vi "Teleop Rollers Control.vi"(9 "Driver Buttons":T1, 10 "Manipulator Axes":T2, 11 "Manipulator Buttons":T1) -> (3 "Roller Command":T3)   [LabVIEW 2013]
uses:
  <vilib>/Rock Robotics/WPI/Joystick/WPI_JoystickButtonState.ctl
  Roller Control.ctl
  Roller Mode.ctl
  Common Code/Change Detect Boolean.vi
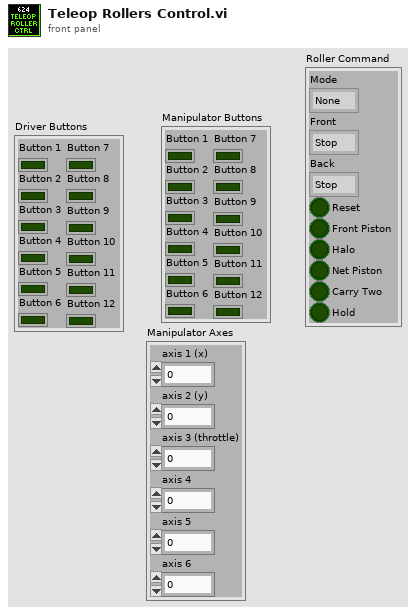
[diagram p1: front panel]
types:
  T1 = typedef "WPI_JoystickButtonState.ctl" = cluster{"Button 1":bool, "Button 2":bool, "Button 3":bool, "Button 4":bool, "Button 5":bool, "Button 6":bool, "Button 7":bool, "Button 8":bool, "Button 9":bool, "Button 10":bool, "Button 11":bool, "Button 12":bool}
  T2 = cluster{"axis 1 (x)":dbl, "axis 2 (y)":dbl, "axis 3 (throttle)":dbl, "axis 4":dbl, "axis 5":dbl, "axis 6":dbl}
  T3 = typedef "Roller Control.ctl" = cluster{"Mode":T4, "Front":enum16{"Stop", "Forward", "Reverse"}, "Back":enum16{"Stop", "Forward", "Reverse"}, "Reset":bool, "Front Piston":bool, "Halo":bool, "Net Piston":bool, "Carry Two":bool, "Hold":bool}
  T4 = typedef "Roller Mode.ctl" = enum16{"None", "Front", "Back", "Both", "Manual"}
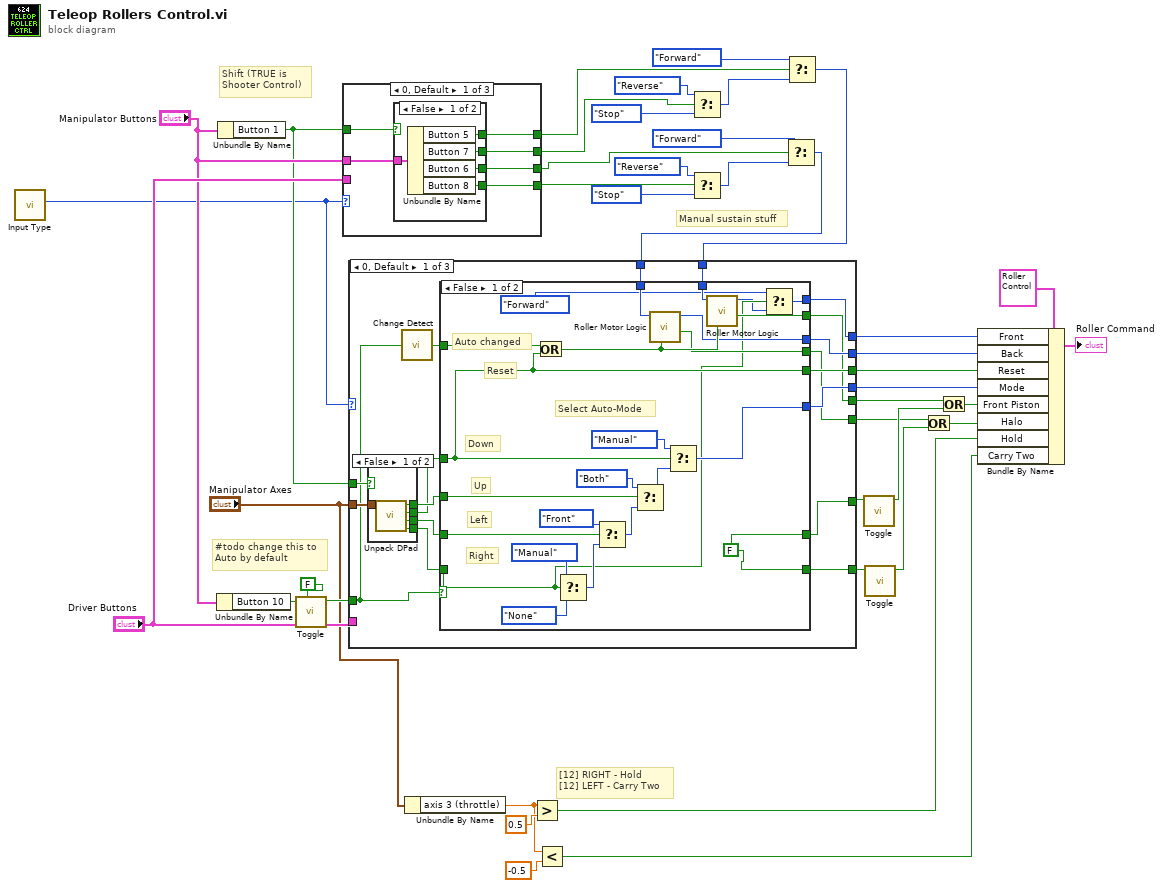
[diagram p0: block diagram]
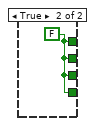
[diagram p2: hidden frame]
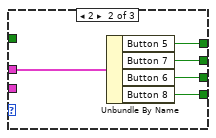
[diagram p3: hidden frame]
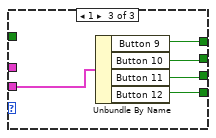
[diagram p4: hidden frame]
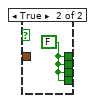
[diagram p5: hidden frame]
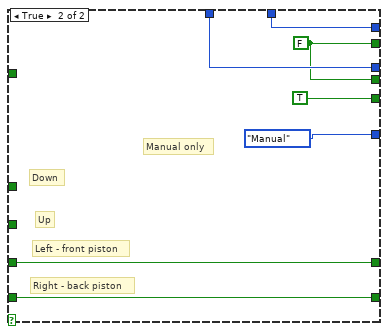
[diagram p6: hidden frame]
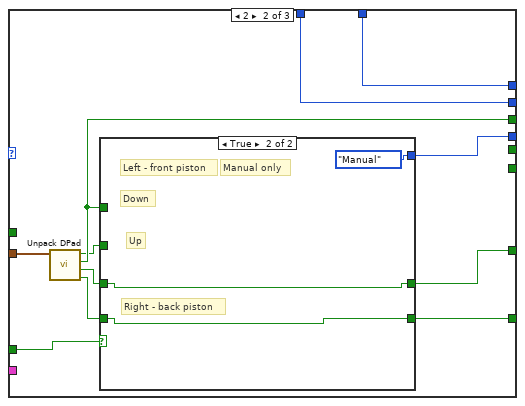
[diagram p7: hidden frame]
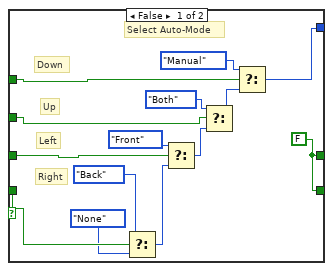
[diagram p8: hidden frame]
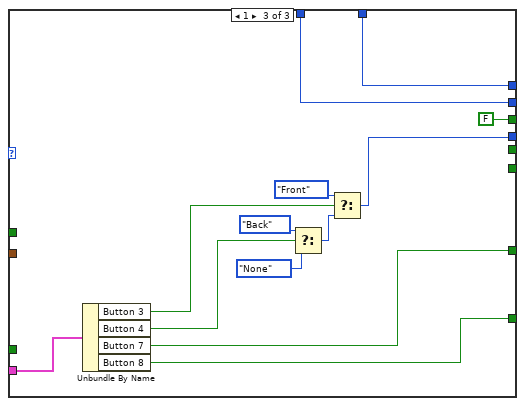
[diagram p9: hidden frame]
diagram:
  # "Manual sustain stuff"
  # "[12] RIGHT - Hold\n[12] LEFT - Carry Two"
  # "Shift (TRUE is\nShooter Control)"
  # "#todo change this to\nAuto by default"
  n1 = call "Input Type.vi"() -> ("Mode"=w17:i32)  [unwired: 11 in]
  n2 = Unbundle By Name("Manipulator Buttons") -> ("Button 10"=w27:bool)
  n3 = Unbundle By Name("Manipulator Buttons") -> ("Button 1"=w18:bool)
  n4 = call "Toggle.vi"("Initial Value"=FALSE, "In"=w27) -> ("Toggled"=w28:bool)  [unwired: 9 in]
  n5 = case shown="0, Default" w17 {
    tunnel: [w44 w55 w59] -> w32
    tunnel: [w45 w56 w60] -> w21
    tunnel: [w46 w57 w61] -> w22
    tunnel: [w47 w58 w62] -> w23
    tunnel: "Manipulator Buttons" -> [w43 w54 _]
    tunnel: "Driver Buttons" -> [_ _ w63]
    tunnel: w18 -> [w42 _ _]
    frame 0, Default {
      n6 = case shown="False" w42 {
        tunnel: [w52 w53] -> w47
        tunnel: [w51 w53] -> w46
        tunnel: [w50 w53] -> w45
        tunnel: [w49 w53] -> w44
        tunnel: w43 -> [w48 _]
        frame False {
          n7 = Unbundle By Name(w48) -> ("Button 5"=w52:bool, "Button 7"=w51:bool, "Button 6"=w50:bool, "Button 8"=w49:bool)
        }
        frame True {
          w53 = FALSE ("Button 5")
        }
      }
    }
    frame 2 {
      n8 = Unbundle By Name(w54) -> ("Button 5"=w58:bool, "Button 7"=w57:bool, "Button 6"=w56:bool, "Button 8"=w55:bool)
    }
    frame 1 {
      n9 = Unbundle By Name(w63) -> ("Button 9"=w62:bool, "Button 10"=w61:bool, "Button 11"=w60:bool, "Button 12"=w59:bool)
    }
  }
  n10 = Unbundle By Name("Manipulator Axes") -> ("axis 3 (throttle)"=w2:dbl)
  n11 = Greater?(x=w2, y=0.5) -> (0:w14:bool)
  n12 = Less?(x=w2, y=-0.5) -> (x < y?=w1:bool)
  n13 = Select(t=enum16{"Stop", "Forward", "Reverse"}."Reverse" ("Front"), s=w22, f=enum16{"Stop", "Forward", "Reverse"}."Stop" ("Front")) -> (s? t:f=w34:enum16{"Stop", "Forward", "Reverse"})
  n14 = Select(t=enum16{"Stop", "Forward", "Reverse"}."Reverse" ("Front"), s=w32, f=enum16{"Stop", "Forward", "Reverse"}."Stop" ("Front")) -> (s? t:f=w38:enum16{"Stop", "Forward", "Reverse"})
  n15 = Select(t=enum16{"Stop", "Forward", "Reverse"}."Forward" ("Front"), s=w21, f=w38) -> (s? t:f=w13:enum16{"Stop", "Forward", "Reverse"})
  n16 = Select(t=enum16{"Stop", "Forward", "Reverse"}."Forward" ("Front"), s=w23, f=w34) -> (s? t:f=w12:enum16{"Stop", "Forward", "Reverse"})
  n17 = case shown="0, Default" w17 {
    tunnel: w28 -> [w67 w126 _]
    tunnel: [w81 w129 w155] -> w30
    tunnel: "Manipulator Axes" -> [w75 w121 _]
    tunnel: [w72 w123 FALSE ("Toggled")] -> w29
    tunnel: "Driver Buttons" -> [_ _ w158]
    tunnel: [w80 w127 w152] -> w25
    tunnel: [w79 w128 w153] -> w20
    tunnel: w18 -> [w74 _ _]
    tunnel: w13 -> [w69 w119 w147]
    tunnel: w12 -> [w71 w120 w148]
    tunnel: [w70 w120 w148] -> w11
    tunnel: [w68 w119 w147] -> w10
    tunnel: [w65 _ _] -> w5
    tunnel: [w64 _ _] -> w4
    frame 0, Default {
      n18 = case shown="False" w74 {
        tunnel: [w86 w87] -> w78
        tunnel: [w85 w87] -> w77
        tunnel: [w84 w87] -> w73
        tunnel: [w83 w87] -> w76
        tunnel: w75 -> [w82 _]
        frame False {
          n19 = call "Unpack DPad.vi"("Axes"=w82) -> ("Right"=w86:bool, "Left"=w85:bool, "Down"=w84:bool, "Up"=w83:bool)  [unwired: 7 in]
        }
        frame True {
          w87 = FALSE ("Up")
        }
      }
      n20 = call-poly "Change Detect.vi"("In"=w67) -> ("Changed?"=w66:bool)
      n21 = case shown="False" w67 {
        tunnel: [w107 Roller_Mode."Manual" ("Roller Mode")] -> w81
        tunnel: w76 -> [w110 _]
        tunnel: w73 -> [w98 _]
        tunnel: w77 -> [w92 w118]
        tunnel: w78 -> [w91 w117]
        tunnel: [w106 w118] -> w79
        tunnel: [w106 w117] -> w80
        tunnel: [w98 TRUE ("Up")] -> w72
        tunnel: w71 -> [w100 w114]
        tunnel: [w89 w114] -> w70
        tunnel: w69 -> [w99 w113]
        tunnel: [w95 w113] -> w68
        tunnel: w66 -> [w96 _]
        tunnel: [w94 w112] -> w65
        tunnel: [w93 w112] -> w64
        frame False {
          w106 = FALSE ("Left")
          # "Reset"
          # "Auto changed"
          # "Left"
          # "Up"
          # "Down"
          # "Select Auto-Mode"
          # "Right"
          n22 = Or(x=w96, y=w98) -> (x .or. y?=w97:bool)
          n23 = Select(t=Roller_Mode."Manual" ("Roller Mode"), s=w91, f=Roller_Mode."None" ("Roller Mode")) -> (s? t:f=w111:T4)
          n24 = Select(t=Roller_Mode."Front" ("Roller Mode"), s=w92, f=w111) -> (s? t:f=w109:T4)
          n25 = Select(t=Roller_Mode."Both" ("Roller Mode"), s=w110, f=w109) -> (s? t:f=w108:T4)
          n26 = call "Roller Motor Logic.vi"("Reset?"=w97, "Command in"=w99) -> ("Solenoid out"=w93:bool, "Command out"=w95:enum16{"Stop", "Forward", "Reverse"})  [unwired: 8 in]
          n27 = Select(t=Roller_Mode."Manual" ("Roller Mode"), s=w98, f=w108) -> (s? t:f=w107:T4)
          n28 = call "Roller Motor Logic.vi"("Reset?"=w97, "Command in"=w100) -> ("Solenoid out"=w94:bool, "Command out"=w90:enum16{"Stop", "Forward", "Reverse"})  [unwired: 8 in]
          n29 = Select(t=enum16{"Stop", "Forward", "Reverse"}."Forward", s=w91, f=w90) -> (s? t:f=w89:enum16{"Stop", "Forward", "Reverse"})
        }
        frame True {
          w112 = FALSE ("Solenoid out")
          # "Left - front piston"
          # "Up"
          # "Down"
          # "Right - back piston"
          # "Manual only"
        }
      }
    }
    frame 2 {
      n30 = call "Unpack DPad.vi"("Axes"=w121) -> ("Right"=w125:bool, "Left"=w124:bool, "Down"=w123:bool, "Up"=w122:bool)  [unwired: 7 in]
      n31 = case shown="True" w126 {
        tunnel: [w138 Roller_Mode."Manual" ("Roller Mode")] -> w129
        tunnel: w122 -> [w143 _]
        tunnel: w123 -> [w141 _]
        tunnel: w124 -> [w142 w146]
        tunnel: w125 -> [w140 w145]
        tunnel: [w139 w146] -> w128
        tunnel: [w139 w145] -> w127
        frame False {
          w139 = FALSE ("Left")
          # "Left"
          # "Right"
          # "Up"
          # "Down"
          # "Select Auto-Mode"
          n32 = Select(t=Roller_Mode."Back" ("Roller Mode"), s=w140, f=Roller_Mode."None" ("Roller Mode")) -> (s? t:f=w135:T4)
          n33 = Select(t=Roller_Mode."Front" ("Roller Mode"), s=w142, f=w135) -> (s? t:f=w136:T4)
          n34 = Select(t=Roller_Mode."Both" ("Roller Mode"), s=w143, f=w136) -> (s? t:f=w137:T4)
          n35 = Select(t=Roller_Mode."Manual" ("Roller Mode"), s=w141, f=w137) -> (s? t:f=w138:T4)
        }
        frame True {
          # "Left - front piston"
          # "Manual only"
          # "Down"
          # "Right - back piston"
          # "Up"
        }
      }
    }
    frame 1 {
      n36 = Unbundle By Name(w158) -> ("Button 3"=w156:bool, "Button 4"=w157:bool, "Button 7"=w153:bool, "Button 8"=w152:bool)
      n37 = Select(t=Roller_Mode."Back" ("Roller Mode"), s=w157, f=Roller_Mode."None" ("Roller Mode")) -> (s? t:f=w159:T4)
      n38 = Select(t=Roller_Mode."Front" ("Roller Mode"), s=w156, f=w159) -> (s? t:f=w155:T4)
    }
  }
  n39 = call "Toggle.vi"("In"=w20) -> ("Toggled"=w9:bool)  [unwired: 10 in]
  n40 = call "Toggle.vi"("In"=w25) -> ("Toggled"=w7:bool)  [unwired: 10 in]
  n41 = Or(x=w4, y=w7) -> (x .or. y?=w6:bool)
  n42 = Or(x=w5, y=w9) -> (x .or. y?=w8:bool)
  n43 = Bundle By Name(cluster=T3 {"Mode"=enum."None", "Front"=enum."Stop", "Back"=enum."Stop", "Reset"=FALSE, "Front Piston"=FALSE, "Halo"=FALSE, "Net Piston"=FALSE, "Carry Two"=FALSE, "Hold"=FALSE} ("Roller Command"), "Front"=w11, "Back"=w10, "Reset"=w29, "Mode"=w30, "Front Piston"=w8, "Halo"=w6, "Hold"=w14, "Carry Two"=w1) -> (→"Roller Command":T3)
